vi "5492_WPI_RobotDriveOpen6MotorWithTalonSRXPosition.vi"(0 "Front Left Motor":T1=enum."Invalid", 1 "Front Right Motor":T1=enum."Invalid", 2 "Back Left Motor":T1=enum."Invalid", 3 "Back Right Motor":T1=enum."Invalid", 4 "Middle Left Motor":T1=enum."Invalid", 5 "Middle Right Motor":T1=enum."Invalid", 7 "error in (no error)":errorcluster, 8 "Front Left Motor Inverted":bool, 9 "Middle Left Motor Inverted":bool, 10 "Back Left Motor Inverted":bool, 15 "Back Right Motor Inverted":bool, 16 "Front Right Motor Inverted":bool, 17 "Middle Right Motor Inverted":bool) -> (20 "RobotDriveDevRef":T2={"DevStatus"={"status"=FALSE, "code"=0, "source"=""}, "Motors[]"=[], "Square Inputs"=FALSE, "Max Output"=1.0}, 27 "error out":errorcluster)   [LabVIEW 2016]
doc: "Opens a reference to the robot drive for a two-motor robot using TalonSRX motor controllers.\n\nThis software is licensed. Open the labview\\readme\\WPI Robotics Library Open Source License.txt file for more information."
uses:
  <vilib>/Rock Robotics/SystemInterfaces/DIO/FPGA_DIOPWMChannel.ctl
  <vilib>/Rock Robotics/WPI/RobotDrive/WPI_RobotDriveDevRef.ctl
  <vilib>/Rock Robotics/WPI/MotorControl/WPI_MotorControlDeviceRef.ctl
  <vilib>/Rock Robotics/WPI/MotorControl/WPI_MotorControlType.ctl
  <vilib>/Rock Robotics/WPI/PWM/WPI_PWMDeadband.ctl
  <vilib>/Rock Robotics/WPI/SafetyOutput/WPI_SafetyOutputConfigMenu.ctl
  <vilib>/Rock Robotics/WPI/ThirdParty/CanMotor/TalonSRX/WPI_CANTalonSRX_APIControlMode.ctl
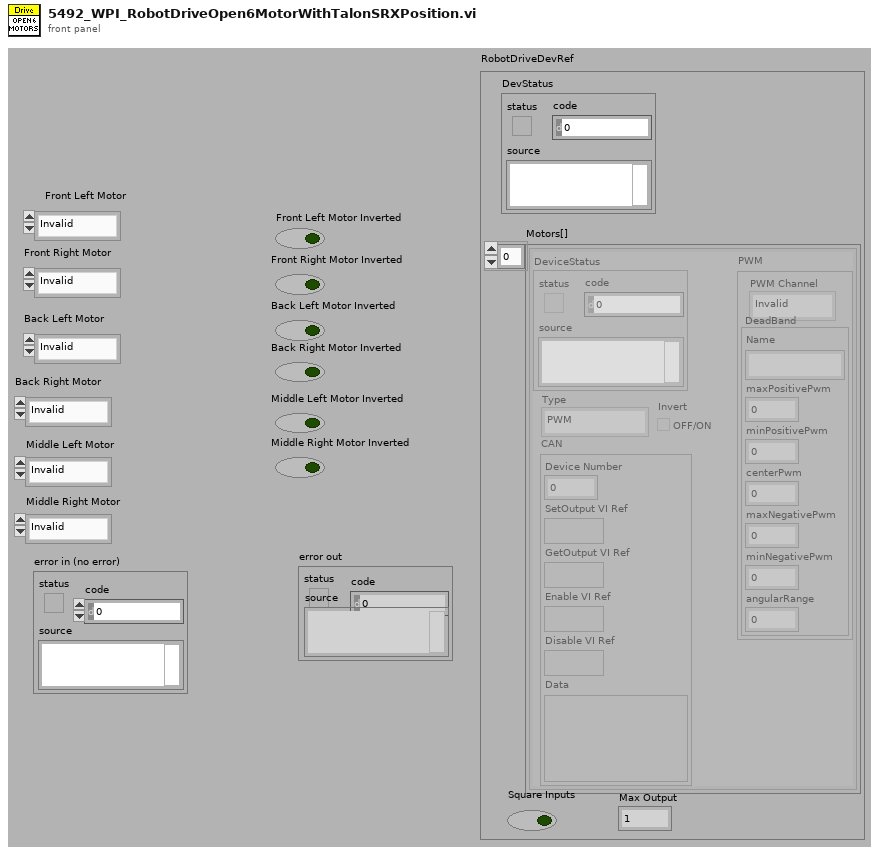
[diagram p1: front panel]
types:
  T1 = typedef "FPGA_DIOPWMChannel.ctl" = enum8{"PWM 0", "PWM 1", "PWM 2", "PWM 3", "PWM 4", "PWM 5", "PWM 6", "PWM 7", "PWM 8", "PWM 9", "PWM MXP 0", "PWM MXP 1", "PWM MXP 2", "PWM MXP 3", "PWM MXP 4", "PWM MXP 5", "PWM MXP 6", "PWM MXP 7", "PWM MXP 8", "PWM MXP 9", "Invalid"}
  T2 = typedef "WPI_RobotDriveDevRef.ctl" = cluster{"DevStatus":errorcluster, "Motors[]":T3[], "Square Inputs":bool, "Max Output":dbl}
  T3 = typedef "WPI_MotorControlDeviceRef.ctl" = cluster{"DeviceStatus":errorcluster, "Type":T4, "PWM":cluster{"PWM Channel":T1, "DeadBand":T5}, "CAN":cluster{"Device Number":u8, "SetOutput VI Ref":variant, "GetOutput VI Ref":variant, "Enable VI Ref":variant, "Disable VI Ref":variant, "Data":variant}, "Invert":bool}
  T4 = typedef "WPI_MotorControlType.ctl" = enum16{"PWM", "CAN"}
  T5 = typedef "WPI_PWMDeadband.ctl" = cluster{"Name":string, "maxPositivePwm":i32, "minPositivePwm":i32, "centerPwm":i32, "maxNegativePwm":i32, "minNegativePwm":i32, "angularRange":u16}
  T6 = typedef "WPI_CANTalonSRX_APIControlMode.ctl" = enum8{"Percent VBus", "Speed", "Position", "Slave", "Unchanged / Invalid", "Voltage Compensation", "Current", "Motion Profile", "Motion Magic"}
  T7 = typedef "WPI_SafetyOutputConfigMenu.ctl" = enum16{"Enable", "Disable"}
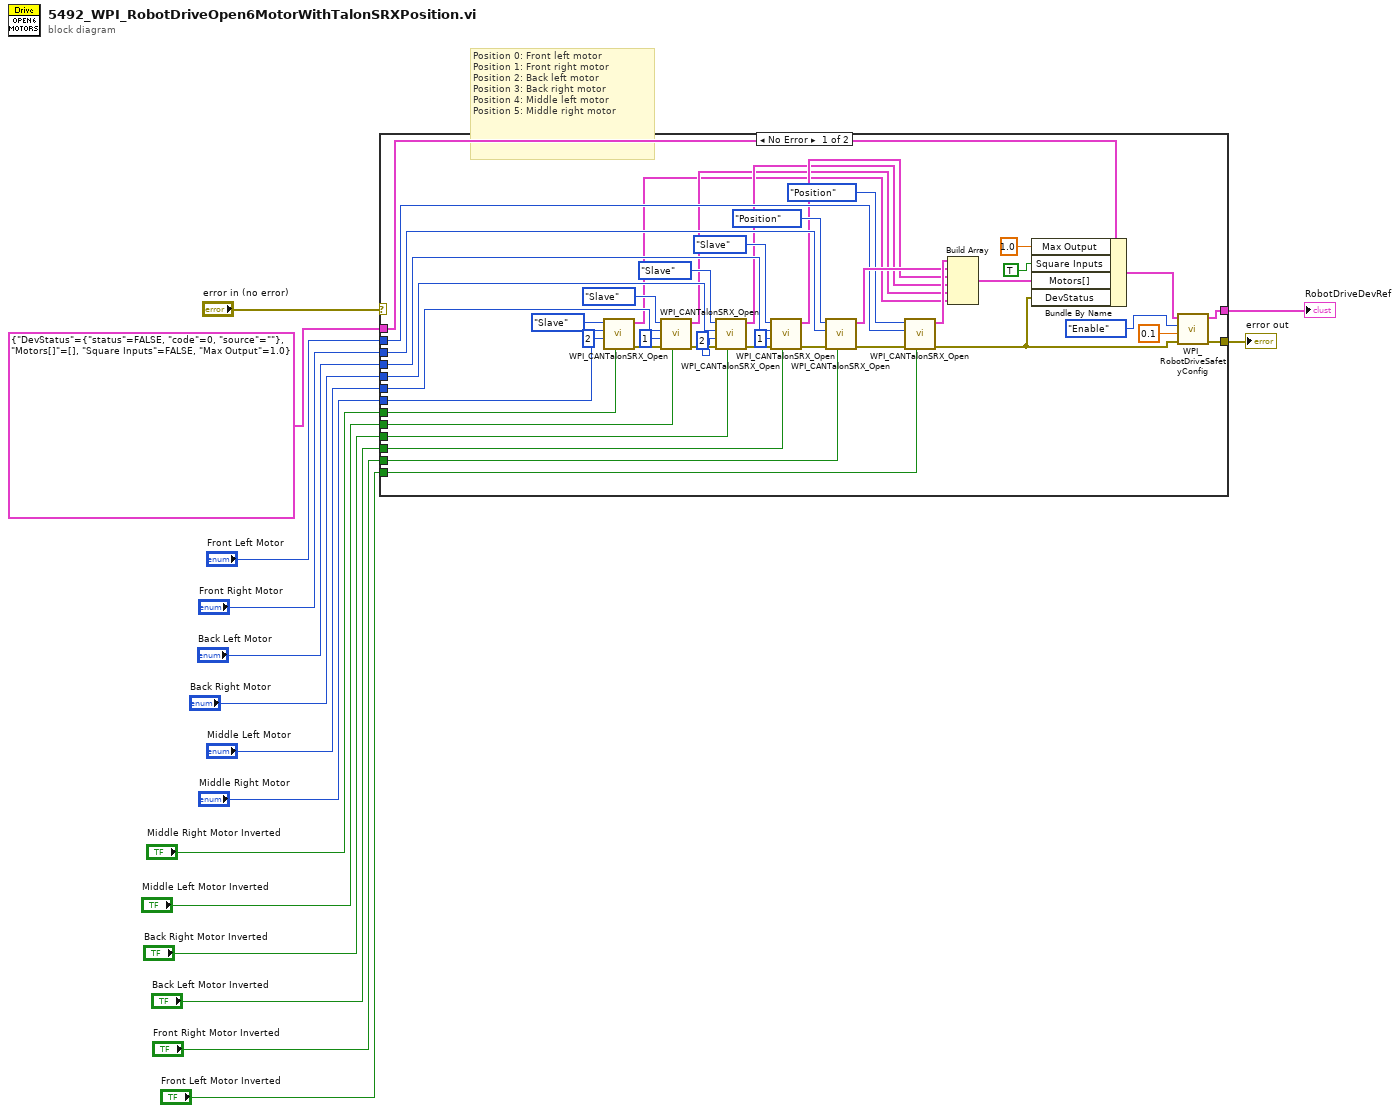
[diagram p0: block diagram]
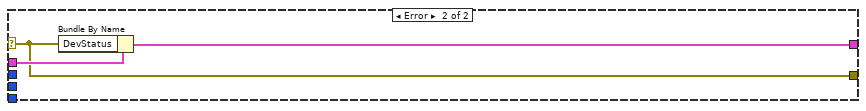
[diagram p2: hidden frame]
diagram:
  # "Position 0: Front left motor\nPosition 1: Front right motor\nPosition 2: Back left motor\nPosition 3: Back right motor\nPosition 4: Middle left motor\nPosition 5: Middle right motor"
  n1 = case shown="No Error" "error in (no error)" {
    selector: "error in (no error)" -> [_ w60]
    tunnel: "Front Left Motor" -> [w41 _]
    tunnel: "Front Right Motor" -> [w39 _]
    tunnel: [w47 w62] -> w9
    tunnel: "Front Left Motor Inverted" -> [w53 _]
    tunnel: "Front Right Motor Inverted" -> [w54 _]
    tunnel: T2 {"DevStatus"={"status"=FALSE, "code"=0, "source"=""}, "Motors[]"=[], "Square Inputs"=FALSE, "Max Output"=1.0} ("RobotDriveDevRef") -> [w58 w61]
    tunnel: [w48 w60] -> w11
    tunnel: "Middle Left Motor" -> [w37 _]
    tunnel: "Middle Right Motor" -> [w35 _]
    tunnel: "Middle Left Motor Inverted" -> [w44 _]
    tunnel: "Middle Right Motor Inverted" -> [w43 _]
    tunnel: "Back Left Motor" -> [w31 _]
    tunnel: "Back Left Motor Inverted" -> [w30 _]
    tunnel: "Back Right Motor" -> [w29 _]
    tunnel: "Back Right Motor Inverted" -> [w28 _]
    frame No Error {
      n2 = call <vilib>:"WPI_CANTalonSRX_Open.vi"("Invert"=w43, "Master Device Number"=u8 2, "Device Number"=w35, "Control Mode"=WPI_CANTalonSRX_APIControlMode."Slave") -> ("error out"=w42:errorcluster, "CAN Talon SRX Ref"=w21:T3)  [unwired: 6 in]
      n3 = call <vilib>:"WPI_CANTalonSRX_Open.vi"("Invert"=w44, "error in"=w42, "Master Device Number"=u8 1, "Device Number"=w37, "Control Mode"=WPI_CANTalonSRX_APIControlMode."Slave") -> ("error out"=w27:errorcluster, "CAN Talon SRX Ref"=w22:T3)  [unwired: 5 in]
      n4 = call <vilib>:"WPI_CANTalonSRX_Open.vi"("Invert"=w28, "error in"=w27, "Master Device Number"=u8 2, "Device Number"=w29, "Control Mode"=WPI_CANTalonSRX_APIControlMode."Slave") -> ("error out"=w26:errorcluster, "CAN Talon SRX Ref"=w23:T3)  [unwired: 5 in]
      n5 = call <vilib>:"WPI_CANTalonSRX_Open.vi"("Invert"=w30, "error in"=w26, "Master Device Number"=u8 1, "Device Number"=w31, "Control Mode"=WPI_CANTalonSRX_APIControlMode."Slave") -> ("error out"=w25:errorcluster, "CAN Talon SRX Ref"=w24:T3)  [unwired: 5 in]
      n6 = call <vilib>:"WPI_CANTalonSRX_Open.vi"("Invert"=w54, "error in"=w25, "Device Number"=w39, "Control Mode"=WPI_CANTalonSRX_APIControlMode."Position") -> ("error out"=w57:errorcluster, "CAN Talon SRX Ref"=w55:T3)  [unwired: 6 in]
      n7 = call <vilib>:"WPI_CANTalonSRX_Open.vi"("Invert"=w53, "error in"=w57, "Device Number"=w41, "Control Mode"=WPI_CANTalonSRX_APIControlMode."Position") -> ("error out"=w49:errorcluster, "CAN Talon SRX Ref"=w56:T3)  [unwired: 6 in]
      n8 = Build Array(w56, w55, w24, w23, w22, w21) -> (w59:T3[])
      n9 = Bundle By Name(cluster=w58, "Max Output"=1.0, "Square Inputs"=TRUE, "Motors[]"=w59, "DevStatus"=w49) -> (w51:T2)
      n10 = call <vilib>:"WPI_RobotDriveSafetyConfig.vi"("error in (no error)"=w49, "timeout (s)"=0.1, "mode"=WPI_SafetyOutputConfigMenu."Enable", "RobotDriveDevRef"=w51) -> ("error out"=w48:errorcluster, "RobotDriveDevRef"=w47:T2)  [unwired: 6 out]
    }
    frame Error {
      n11 = Bundle By Name(cluster=w61, "DevStatus"=w60) -> (w62:T2)
    }
  }
  "RobotDriveDevRef" <- w9
  "error out" <- w11
